vi "SpkCycle.vi"(7 "LabVIEW Web Service Request":refnum<class "Web Request.lvclass">, 9 "length":i16, 10 "period":i16, 11 "Cycle":u8) -> ()   [LabVIEW 2014]
uses:
  <vilib>/wsapi/Web Request.lvclass
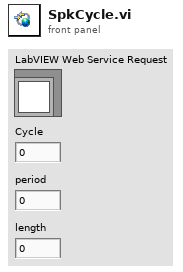
[diagram p1: front panel]
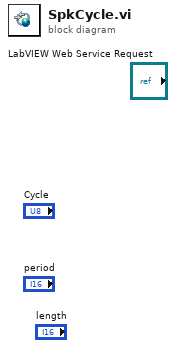
[diagram p0: block diagram]
diagram:
